vi "processScanCommand.vi"(0 "FPGA VI Reference In":T5, 5 "Queues":T6, 9 "scale factors (um/level)":dbl[](array[numeric])=[0.016, 0.016, 0.00025], 11 "error in (no error)":errorcluster, 12 "tracker status":T1) -> (1 "line volume nums":i32[](array[numeric]), 3 "num new volumes":i32, 4 "num calls":T4, 6 "current volume":T3, 8 "command queue status":T2, 10 "num kalmans per axis":u32[](array[numeric]), 14 "num lines sent":u32, 15 "error out":errorcluster)   [LabVIEW 2010]
uses:
  internal_queues.ctl
  line_info.ctl
  volume_with_lines.ctl
  volume_info.ctl
  kalman_result_scaled.ctl
  projection buffers.ctl
  location3D.ctl
  spot location.ctl
  FPGA_ref.ctl
  tracker status.ctl
  <vilib>/rvi/interface/nirviMethod/nirviMethod.xnode
  <vilib>/rvi/interface/common/niFpgaNodeNameForErrorReporting.ctl
  <vilib>/rvi/errors/niLvFpgaWhatHappensToTopLevelVI.ctl
  FPGA scanInfo/scan message.ctl
  kalman_result_unscaled.ctl
  <vilib>/Utility/error.llb/Error Cluster From Error Code.vi
  <vilib>/rvi/errors/niLvFpgaAdjustHostInterfaceError.vi
  NiFpgaLv.dll
panel:
  # "140 kHz * 2 = 280/ms"
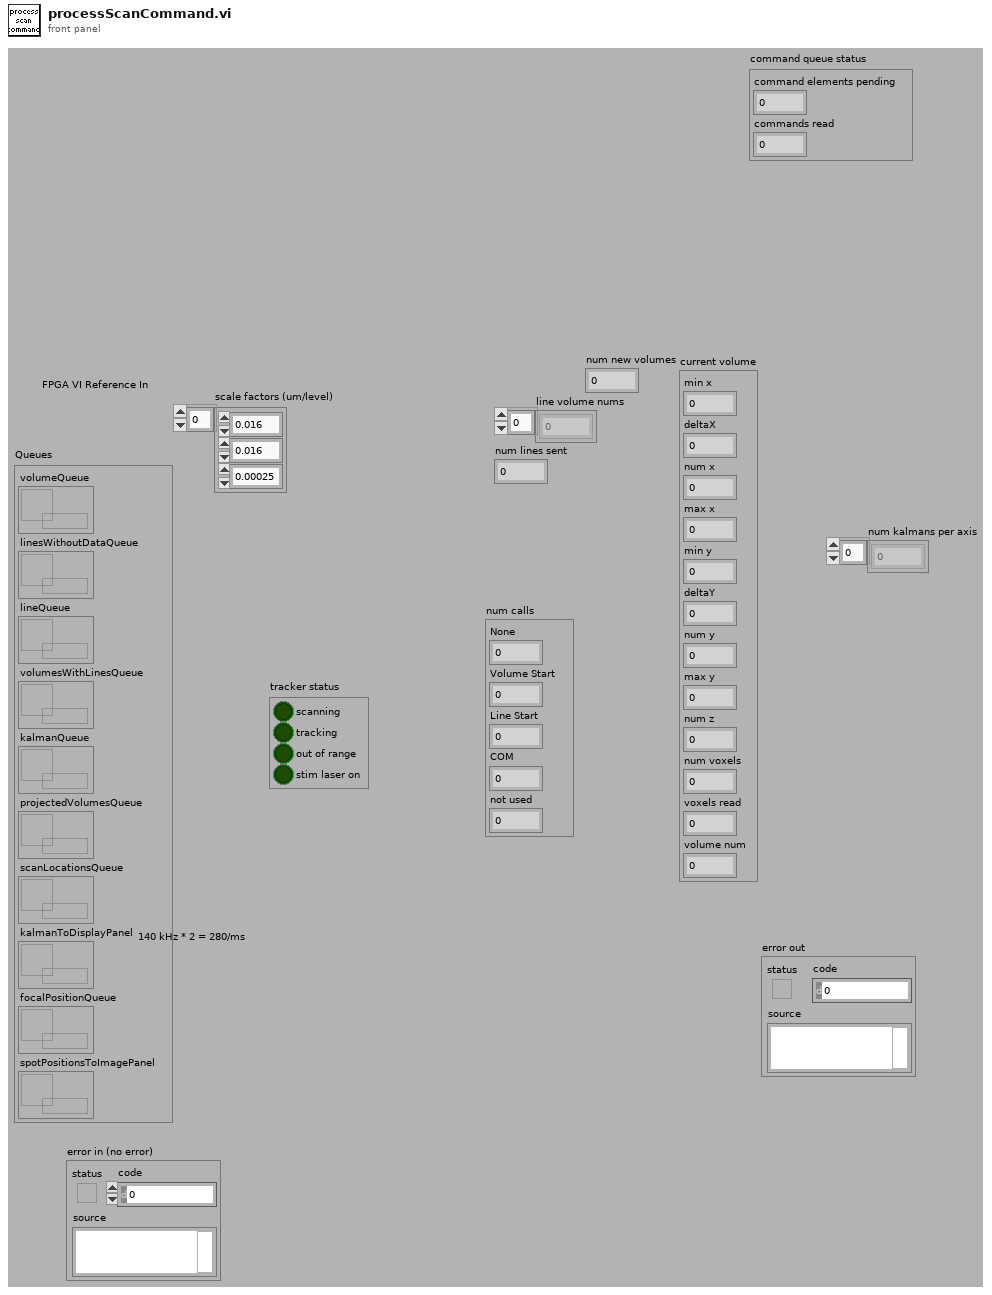
[diagram p1: front panel]
types:
  T1 = typedef "tracker status.ctl" = cluster{"scanning":bool, "tracking":bool, "out of range":bool, "stim laser on":bool}
  T2 = cluster{"command elements pending":u32, "commands read":u32}
  T3 = cluster{"min x":i16, "deltaX":dbl, "num x":u32, "max x":i16, "min y":i16, "deltaY":dbl, "num y":u32, "max y":i16, "num z":u32, "num voxels":u32, "voxels read":u32, "volume num":u32}
  T4 = cluster{"None":i32, "Volume Start":i32, "Line Start":i32, "COM":i32, "not used":i32}
  T5 = typedef "FPGA_ref.ctl" = refnum<k20>
  T6 = typedef "internal_queues.ctl" = cluster{"volumeQueue":refnum<queue>, "linesWithoutDataQueue":refnum<queue>, "lineQueue":refnum<queue>, "volumesWithLinesQueue":refnum<queue>, "kalmanQueue":refnum<queue>, "projectedVolumesQueue":refnum<queue>, "scanLocationsQueue":refnum<queue>, "kalmanToDisplayPanel":refnum<queue>, "focalPositionQueue":refnum<queue>, "spotPositionsToImagePanel":refnum<queue>}
  T7 = cluster{"[0]":i32, "[1]":i32, "[2]":i32, "[3]":i32, "[4]":i32}
  T8 = typedef "line_info.ctl" = cluster{"start X":i16, "start Y":i16, "start Z":i16, "end X":i16, "end Y":i16, "end Z":i16, "num z":u8, "voxel data":u32[], "volume num":u32, "line number":u16, "line type":u16}
  T9 = typedef "kalman_result_unscaled.ctl" = cluster{"axis":u8, "pos":i16, "vel":i16, "wpe or z_piez":i32, "status":u32, "n photon ch 0":u32, "n photon ch 1":u32, "tick count":u32}
  T10 = cluster{"Data[0]":i32, "Data[1]":i32, "Data[2]":i32, "Data[3]":i32, "Data[4]":i32}
  T11 = typedef "scan message.ctl" = enum8{"NONE", "VOLUME START", "LINE START", "LINE START TRACKING", "XKALMAN", "YKALMAN", "ZKALMAN"}
  T12 = typedef "kalman_result_scaled.ctl" = cluster{"axis":u8, "pos":dbl, "vel":dbl, "wpe or z_piezo":dbl, "status":u32, "n photon ch 0":u32, "n photon ch 1":u32, "elapsed time":dbl}
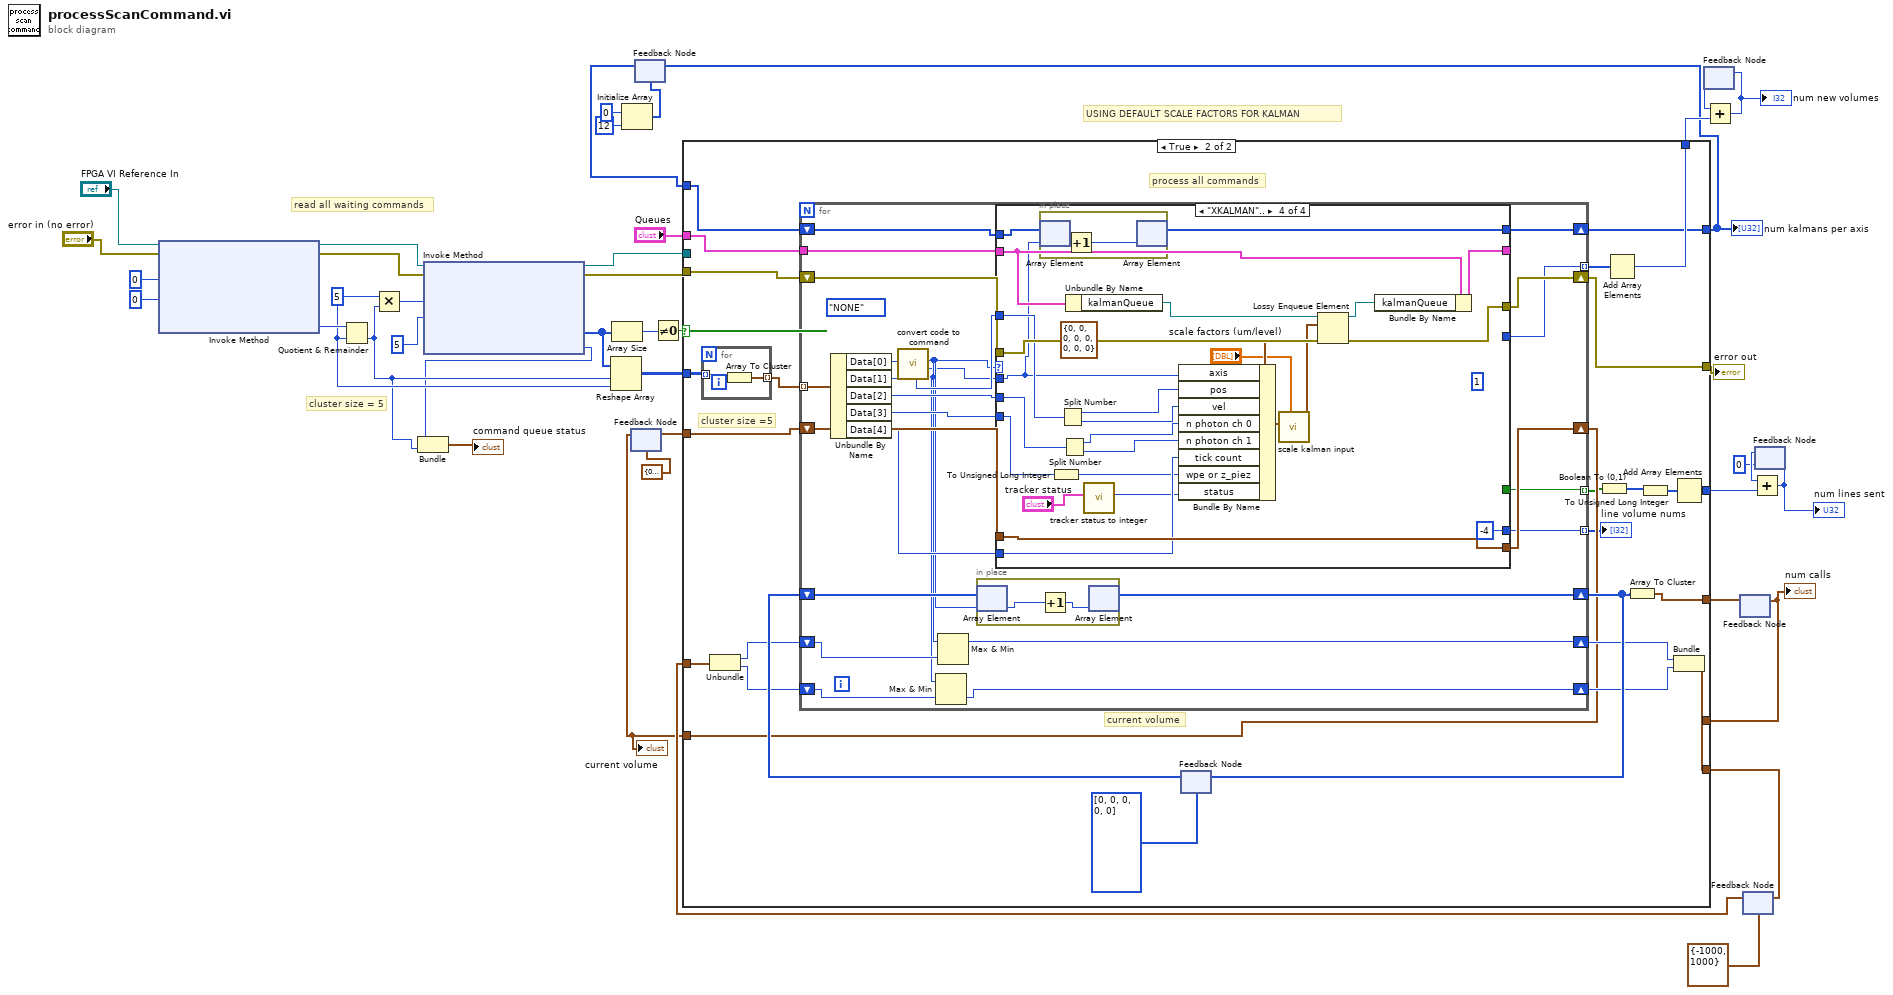
[diagram p0: block diagram]
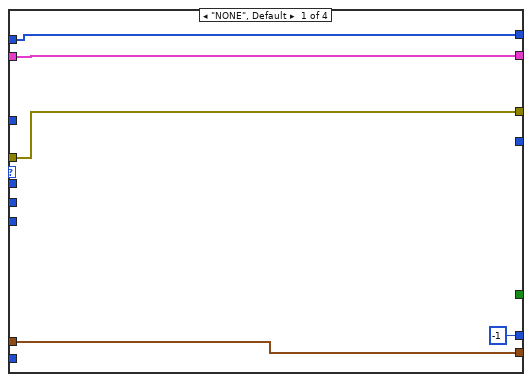
[diagram p3: hidden frame]
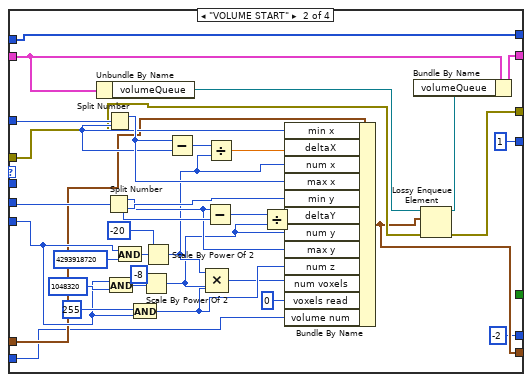
[diagram p4: hidden frame]
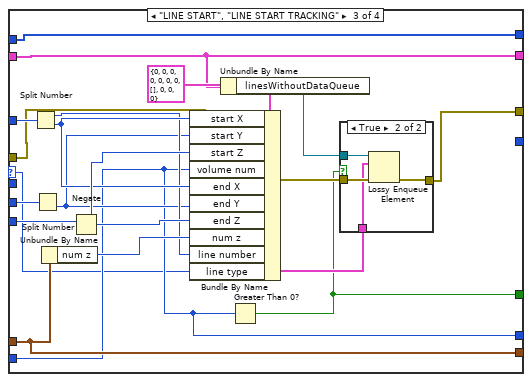
[diagram p5: hidden frame]
diagram:
  w29 = u32 5 ("Number of Elements")
  # "USING DEFAULT SCALE FACTORS FOR KALMAN"
  # "read all waiting commands"
  # "cluster size = 5"
  n1 = xnode "Invoke Method"("FPGA VI Reference In"="FPGA VI Reference In", "error in"="error in (no error)", "Number of Elements"=u32 0, "Timeout (ms)"=0) -> ("FPGA VI Reference Out"=w27:T5, "error out"=w28:errorcluster, "Elements Remaining"=w30:u32)  [unwired: 1 out]
  n2 = Quotient & Remainder(x=w30, y=w29) -> (floor(x/y)=w11:u32)  [unwired: 1 out]
  n3 = Multiply(x=w29, y=w11) -> (x*y=w37:u32)
  n4 = xnode "Invoke Method"("FPGA VI Reference In"=w27, "error in"=w28, "Number of Elements"=w37, "Timeout (ms)"=5) -> ("FPGA VI Reference Out"=w38:T5, "error out"=w39:errorcluster, "Data"=w35:i32[], "Elements Remaining"=w10:u32)
  n5 = Bundle("Elements Remaining"=w10, w11) -> (→"command queue status":cluster{"Elements Remaining":u32, u32})  [unwired: 1 in]
  n6 = Reshape Array(w35, w11, w29) -> (w26:i32[][])
  n7 = Array Size(array=w35) -> (size(s)=w40:i32)
  n8 = Initialize Array(u32 0 ("element"), 12 ("dimension size")) -> (w2:u32[])
  n9 = feedback #1(T3 {"min x"=0, "deltaX"=0.0, "num x"=0, "max x"=0, "min y"=0, "deltaY"=0.0, "num y"=0, "max y"=0, "num z"=0, "num voxels"=0, "voxels read"=0, "volume num"=0} ("current volume")) -> (w14:T3)
  n10 = feedback #2(w2) -> (w1:u32[])
  n11 = Not Equal To 0?(x=w40) -> (x != 0?=w36:bool)
  n12 = feedback #3() -> (w16:i32)  [unwired: 1 in]
  n13 = feedback #4() -> (w22:T7)  [unwired: 1 in]
  "num calls" <- w22
  n14 = feedback #5(cluster{i32, i32} {-1000, 1000}) -> (w21:cluster{i32, i32})
  n15 = case shown="True" w36 {
    tunnel: w39 -> [w46 w72]
    tunnel: w38 -> [_ _]
    tunnel: w26 -> [_ w71]
    tunnel: "Queues" -> [_ w69]
    tunnel: [w46 w54] -> w24
    tunnel: [w45 w65] -> w23
    tunnel: w22 -> [w45 _]
    tunnel: [w44 w62] -> w20
    tunnel: w21 -> [w44 w61]
    tunnel: [_ w57] -> w18
    tunnel: w14 -> [w43 w56]
    tunnel: [w43 w55] -> w13
    tunnel: [_ w49] -> w9
    tunnel: w1 -> [w42 w48]
    tunnel: [w42 w47] -> w3
    frame False {
    }
    frame True {
      # "current volume"
      # "process all commands"
      # "cluster size =5"
      n16 = for {
        tunnel: w71 -> [w192] mode=indexing
        tunnel: [w191] -> w70 mode=indexing
        n17 = Array To Cluster(array=w192) -> (cluster=w191:T10)
      }
      n18 = Unbundle(w61) -> (w60:i32, w59:i32)
      n19 = feedback #6(i32[] [0, 0, 0, 0, 0]) -> (w68:i32[])
      n20 = for {
        tunnel: w70 -> [w80] mode=indexing
        shift-right: [w93] -> w54
        shift-left: w72 -> [w92]
        shift-right: [w90] -> w55
        shift-left: w56 -> [w89]
        shift-right: [w87] -> w66
        shift-left: w68 -> [w88]
        shift-right: [w86] -> w64
        shift-left: w60 -> [w85]
        shift-right: [w84] -> w63
        shift-left: w59 -> [w83]
        tunnel: [w82] -> w58 mode=indexing
        tunnel: w69 -> [w91]
        tunnel: [w79] -> w53 mode=indexing
        tunnel: [w78] -> w52 mode=indexing
        shift-right: [w73] -> w47
        shift-left: w48 -> [w74]
        (unwired) scan_message."NONE" ("Enum")
        n21 = Unbundle By Name(w80) -> ("Data[0]"=w77:i32, "Data[1]"=w96:i32, "Data[2]"=w95:i32, "Data[3]"=w94:i32, "Data[4]"=w81:i32)
        n22 = call "convert code to command.vi"("code"=w77) -> ("axis number"=w75:u8, "command"=w76:T11)  [unwired: 9 in]
        n23 = Max & Min(x=w76, y=w83) -> (min(x,y)=w84:i32)  [unwired: 1 out]
        n24 = Max & Min(x=w76, y=w85) -> (max(x,y)=w86:i32)  [unwired: 1 out]
        n25 = in-place {
          n26 = in-place-array #7(w88, w76) -> (w98:i32)
          n27 = Increment(x=w98) -> (x+1=w97:i32)
          n28 = in-place-array #7(w97) -> (w87:i32[])  [unwired: 1 out]
        }
        n29 = case shown="\"XKALMAN\".." w76 {
          selector: w76 -> [_ _ w140 _]
          tunnel: w96 -> [_ w138 w157 w182]
          tunnel: w95 -> [_ w137 w156 w172]
          tunnel: w94 -> [_ w133 w155 w164]
          tunnel: w91 -> [w103 w119 w150 w188]
          tunnel: w92 -> [w102 w121 w148 w185]
          tunnel: [w103 w117 w150 w187] -> _
          tunnel: [w102 w116 w147 w175] -> w93
          tunnel: [w101 w114 w153 w186] -> w90
          tunnel: w89 -> [w101 w115 w153 w186]
          tunnel: [_ 1 _ _] -> w82
          tunnel: w81 -> [_ w106 w142 w179]
          tunnel: [-1 ("Data[4]") -2 ("Data[4]") w142 -4 ("Data[4]")] -> w79
          tunnel: [_ _ w141 _] -> w78
          tunnel: w75 -> [_ _ _ w166]
          tunnel: w74 -> [w99 w104 w139 w167]
          tunnel: [w99 w104 w139 w165] -> w73
          frame "NONE", Default {
          }
          frame "VOLUME START" {
            n30 = Unbundle By Name(w119) -> ("volumeQueue"=w120:refnum<queue>)
            n31 = Split Number(x=w137) -> (hi(x)=w125:u16, lo(x)=w127:u16)
            n32 = Split Number(x=w138) -> (hi(x)=w130:u16, lo(x)=w129:u16)
            n33 = And(x=w133, y=u32 1048320) -> (x .and. y?=w109:u32)
            n34 = And(x=w133, y=u32 4293918720) -> (x .and. y?=w112:u32)
            n35 = And(x=u32 255, y=w133) -> (x .and. y?=w124:u32)
            n36 = Scale By Power Of 2(n=-8, x=w109) -> (x*2^n=w108:u32)
            n37 = Scale By Power Of 2(n=-20, x=w112) -> (x*2^n=w111:u32)
            n38 = Subtract(x=w130, y=w129) -> (x-y=w132:u16)
            n39 = Subtract(x=w125, y=w127) -> (x-y=w131:u16)
            n40 = Divide(x=w132, y=w111) -> (x/y=w128:dbl)
            n41 = Compound Arithmetic op=MULTIPLY(w111, w108, w124) -> (w123:u32)
            n42 = Divide(x=w131, y=w108) -> (x/y=w126:dbl)
            n43 = Bundle By Name(cluster=w115, "min x"=w129, "deltaX"=w128, "num x"=w111, "max x"=w130, "min y"=w127, "deltaY"=w126, "num y"=w108, "max y"=w125, "num z"=w124, "num voxels"=w123, "voxels read"=u32 0, "volume num"=w106) -> (w114:T3)
            n44 = Lossy Enqueue Element(queue=w120, element=w114, error in (no error)=w121) -> (queue out=w118:refnum<queue>, error out=w116:errorcluster)  [unwired: 2 out]
            n45 = Bundle By Name(cluster=w119, "volumeQueue"=w118) -> (w117:T6)
          }
          frame "LINE START", "LINE START TRACKING" {
            n46 = Split Number(x=w157) -> (hi(x)=w144:u16, lo(x)=w145:u16)
            n47 = Split Number(x=w156) -> (lo(x)=w143:u16)  [unwired: 1 out]
            n48 = Unbundle By Name(w153) -> ("num z"=w152:u32)
            n49 = Negate(x=w155) -> (-x=w154:i32)
            n50 = Bundle By Name(cluster=T8 {"start X"=0, "start Y"=0, "start Z"=0, "end X"=0, "end Y"=0, "end Z"=0, "num z"=0, "voxel data"=[], "volume num"=0, "line number"=0, "line type"=0} ("current line"), "start X"=w145, "start Y"=w143, "start Z"=w155, "volume num"=w142, "end X"=w145, "end Y"=w143, "end Z"=w154, "num z"=w152, "line number"=w144, "line type"=w140) -> (w146:T8)
            n51 = Unbundle By Name(w150) -> ("linesWithoutDataQueue"=w149:refnum<queue>)
            n52 = Greater Than 0?(x=w142) -> (x > 0?=w141:bool)
            n53 = case shown="True" w141 {
              tunnel: w149 -> [_ w162]
              tunnel: w148 -> [w158 w161]
              tunnel: [w158 w160] -> w147
              tunnel: w146 -> [_ w159]
              frame False {
              }
              frame True {
                n54 = Lossy Enqueue Element(queue=w162, element=w159, error in (no error)=w161) -> (error out=w160:errorcluster)  [unwired: 3 out]
              }
            }
          }
          frame "XKALMAN".. {
            (unwired) u32 1
            n55 = in-place {
              n56 = in-place-array #8(w167, w166) -> (w190:u32)
              n57 = Increment(x=w190) -> (x+1=w189:u32)
              n58 = in-place-array #8(w189) -> (w165:u32[])  [unwired: 1 out]
            }
            n59 = To Unsigned Long Integer(number=w164) -> (unsigned 32bit integer=w163:u32)
            n60 = Split Number(x=w182) -> (hi(x)=w181:u16, lo(x)=w180:u16)
            n61 = Split Number(x=w172) -> (hi(x)=w171:u16, lo(x)=w170:u16)
            n62 = Unbundle By Name(w188) -> ("kalmanQueue"=w178:refnum<queue>)
            n63 = call "tracker status to integer.vi"("tracker status"="tracker status") -> ("status integer"=w169:u32)  [unwired: 10 in]
            n64 = Bundle By Name(cluster=T9 {"axis"=0, "pos"=0, "vel"=0, "wpe or z_piez"=0, "status"=0, "n photon ch 0"=0, "n photon ch 1"=0, "tick count"=0} ("kalman result"), "axis"=w166, "pos"=w181, "vel"=w180, "n photon ch 0"=w171, "n photon ch 1"=w170, "tick count"=w179, "wpe or z_piez"=w163, "status"=w169) -> (w176:T9)
            n65 = call "scale kalman input.vi"("x scale factors"="scale factors (um/level)", "kalman result"=w176) -> ("kalman result scaled"=w174:T12)  [unwired: 9 in]
            n66 = Lossy Enqueue Element(queue=w178, element=w174, error in (no error)=w185) -> (queue out=w177:refnum<queue>, error out=w175:errorcluster)  [unwired: 2 out]
            n67 = Bundle By Name(cluster=w188, "kalmanQueue"=w177) -> (w187:T6)
          }
        }
      }
      "line volume nums" <- w53
      n68 = feedback-in #6(w66) -> ()
      n69 = Boolean To (0,1)(Boolean=w52) -> (0, 1=w51:i16[])
      n70 = Add Array Elements(numeric array=w58) -> (sum=w57:i32)
      n71 = Array To Cluster(array=w66) -> (cluster=w65:T7)
      n72 = To Unsigned Long Integer(number=w51) -> (unsigned 32bit integer=w50:u32[])
      n73 = Add Array Elements(numeric array=w50) -> (sum=w49:u32)
      n74 = Bundle(w64, w63) -> (w62:cluster{i32, i32})  [unwired: 1 in]
    }
  }
  "error out" <- w24
  "current volume" <- w13
  "num kalmans per axis" <- w3
  n75 = feedback-in #1(w13) -> ()
  n76 = feedback-in #2(w3) -> ()
  n77 = Add(x=w16, y=w18) -> (x+y=w17:i32)
  "num new volumes" <- w17
  n78 = feedback-in #3(w17) -> ()
  n79 = feedback-in #4(w23) -> ()
  n80 = feedback-in #5(w20) -> ()
  n81 = feedback #9(u32 0) -> (w7:u32)
  n82 = Add(x=w7, y=w9) -> (x+y=w8:u32)
  "num lines sent" <- w8
  n83 = feedback-in #9(w8) -> ()
